vi "CoMP-S TwoCams - Add Error Msg.vi"(8 "error in":errorcluster, 11 "error message (\"\")":string) -> (0 "errorout":errorcluster)   [LabVIEW 2014]
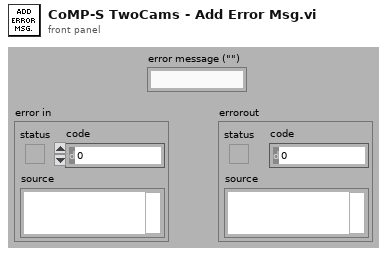
[diagram p1: front panel]
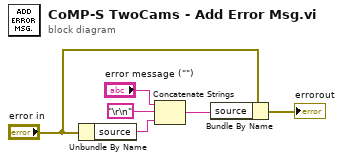
[diagram p0: block diagram]
diagram:
  n1 = Unbundle By Name("error in") -> ("source"=w3:string)
  n2 = Concatenate Strings("error message (\"\")", "\r\n", w3) -> (w5:string)
  n3 = Bundle By Name(cluster="error in", "source"=w5) -> (→"errorout":errorcluster)
